vi "choose code tip.vi"() -> (6 "Python":bool, 10 "Matlab":bool)   [LabVIEW 2010]
panel:
  in  "Python":bool
  in  "Matlab":bool
  # "Select the language:"
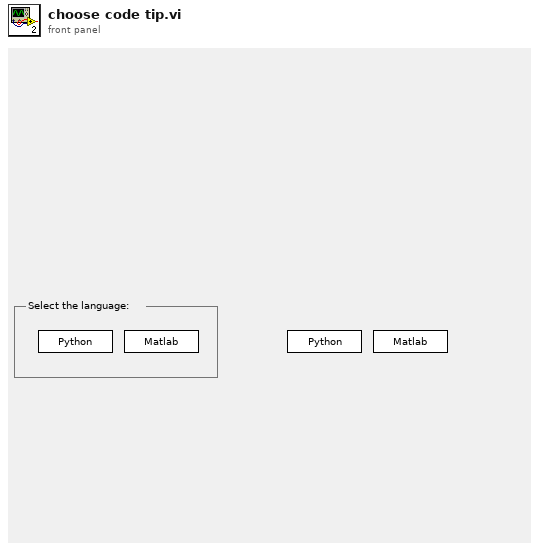
[diagram p1: front panel]
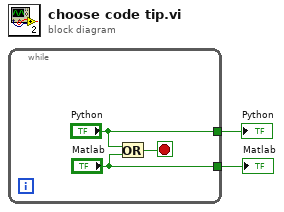
[diagram p0: block diagram]
diagram:
  n1 = while {
    tunnel: ["Matlab"] -> w2
    tunnel: ["Python"] -> w1
    stop <- w5 stop-if-true
    n2 = Or(x="Python", y="Matlab") -> (x .or. y?=w5:bool)
  }
  "Matlab" <- w2
  "Python" <- w1
